vi "Check Status.vi"(8 "error in (no error)":errorcluster, 11 "Analog Output in":refnum<class "Analog Output.lvclass">) -> (0 "error out":errorcluster, 1 "Status":string, 2 "Ready?":bool, 3 "Analog Output out":refnum<class "Analog Output.lvclass">)   [LabVIEW 2017, in "Analog Output.lvclass"]
doc: "(Dynamic) Check if the instrument is powered on and update its member fields with the instrument's current status. Optionally return a text status message."
uses:
  Analog Output.lvclass
  Utility Classes/Scannable/Scannable.lvclass
  <resource>/objmgr/daqmx.rc
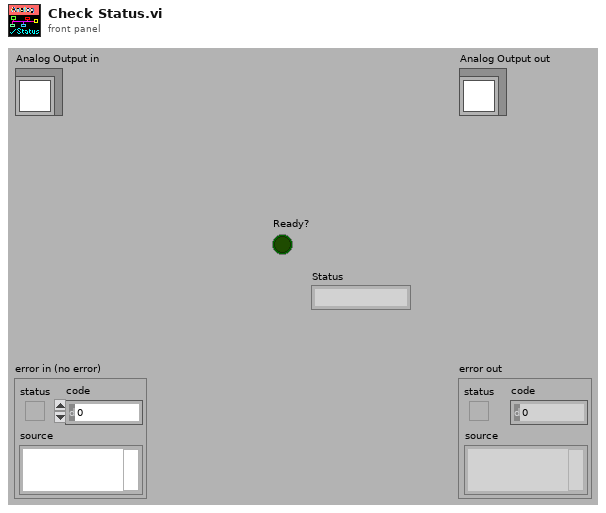
[diagram p1: front panel]
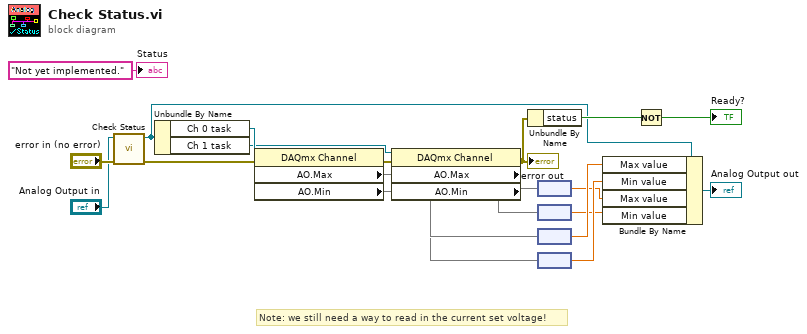
[diagram p0: block diagram]
diagram:
  # "Note: we still need a way to read in the current set voltage!"
  n1 = call-parent "Check Status.vi"("error in (no error)"="error in (no error)", "Instrument in"="Analog Output in") -> ("error out"=w18:errorcluster, "Instrument out"=w5:refnum<class "Analog Output.lvclass">)  [unwired: 6 in, 2 out]
  n2 = Unbundle By Name(w5) -> ("Ch 0 task"=w4:refnum<k21>, "Ch 1 task"=w3:refnum<k21>)
  n3 = property class="DAQmx Channel"(reference=w4, error in=w18) -> (error out=w2:errorcluster, "AO.Max"=w16, "AO.Min"=w14)  [unwired: 1 out]
  n4 = property class="DAQmx Channel"(reference=w3, error in=w2) -> (error out=w1:errorcluster, "AO.Max"=w12, "AO.Min"=w10)  [unwired: 1 out]
  "error out" <- w1
  n5 = Unbundle By Name(w1) -> ("status"=w8:bool)
  n6 = node(w12) -> (w11:dbl[unit])
  n7 = node(w10) -> (w9:dbl[unit])
  n8 = node(w16) -> (w15:dbl[unit])
  n9 = node(w14) -> (w13:dbl[unit])
  n10 = Bundle By Name(cluster=w5, "Max value"=w15, "Min value"=w13, "Max value"=w11, "Min value"=w9) -> (→"Analog Output out":refnum<class "Analog Output.lvclass">)
  n11 = Not(x=w8) -> (.not. x?=→"Ready?":bool)
  "Status" <- "Not yet implemented." ("Status")
